vi "PH_GUI.set U32 ring GUI object.vi"(1 "Strings And Values [Empty]":T2, 2 "Ring Ref":refnum<vi>, 3 "Value":u32, 4 "Blinking (false)":bool, 5 "error in (no error)":errorcluster, 7 "Tip Strip [Empty]":string, 9 "Disabled (Enabled)":T1(ring), 11 "Visible (true)":bool=TRUE) -> (19 "error out":errorcluster)   [LabVIEW 2014, in "PH_Common.lvlib"]
doc: "Sets value and more for the referenced GUI object."
uses:
  <vilib>/Utility/miscctls.llb/LVStringsAndValuesArrayTypeDef_U32.ctl
  PH_Common.lvlib
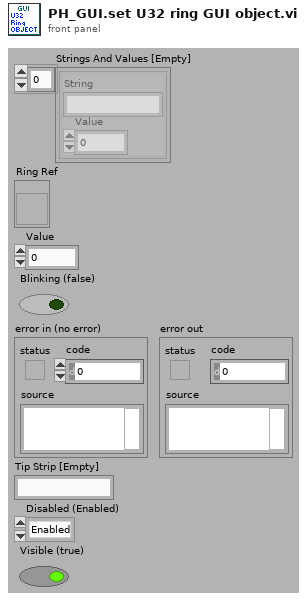
[diagram p1: front panel]
types:
  T1 = enum8{"Enabled", "Disabled", "Disabled and Grayed Out"}
  T2 = typedef "LVStringsAndValuesArrayTypeDef_U32.ctl" = cluster{"String":string, "Value":u32}[]
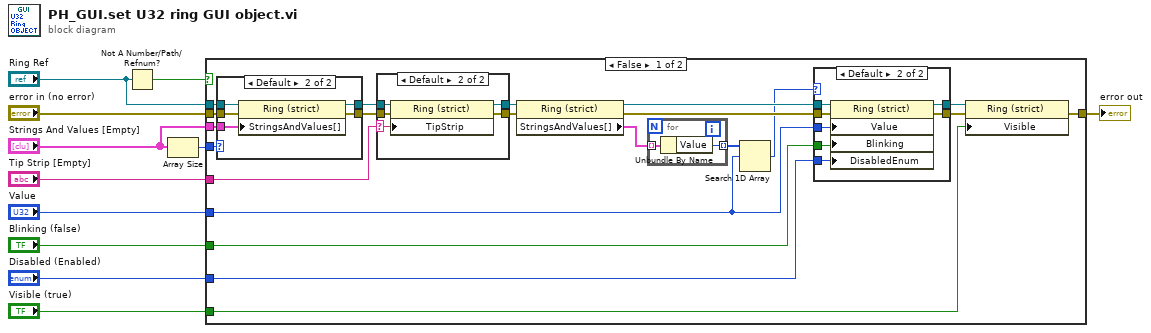
[diagram p0: block diagram]
diagram:
  n1 = Not A Number/Path/Refnum?(number/path/refnum="Ring Ref") -> (NaN/Path/Refnum?=w10:bool)
  n2 = Array Size(array="Strings And Values [Empty]") -> (size(s)=w5:i32)
  n3 = case shown="False" w10 {
    tunnel: "error in (no error)" -> [w24 w58]
    tunnel: "Ring Ref" -> [w25 _]
    tunnel: "Value" -> [w27 _]
    tunnel: "Blinking (false)" -> [w32 _]
    tunnel: [w15 w58] -> w7
    tunnel: w5 -> [w23 _]
    tunnel: "Strings And Values [Empty]" -> [w22 _]
    tunnel: "Tip Strip [Empty]" -> [w17 _]
    tunnel: "Disabled (Enabled)" -> [w16 _]
    tunnel: "Visible (true)" -> [w12 _]
    frame False {
      n4 = case shown="Default" w23 {
        tunnel: w25 -> [w41 w46]
        tunnel: [w41 w45] -> w21
        tunnel: w24 -> [w40 w44]
        tunnel: [w40 w43] -> w19
        tunnel: w22 -> [_ w42]
        frame 0 {
        }
        frame Default {
          n5 = property class="Ring (strict)"(reference=w46, error in=w44, "StringsAndValues[]"=w42) -> (reference out=w45:refnum<vi>, error out=w43:errorcluster)
        }
      }
      n6 = case shown="Default" w17 {
        selector: w17 -> [_ w35]
        tunnel: w21 -> [w34 w39]
        tunnel: [w34 w38] -> w20
        tunnel: w19 -> [w33 w37]
        tunnel: [w33 w36] -> w18
        frame "", "N/A" {
        }
        frame Default {
          n7 = property class="Ring (strict)"(reference=w39, error in=w37, "TipStrip"=w35) -> (reference out=w38:refnum<vi>, error out=w36:errorcluster)
        }
      }
      n8 = property class="Ring (strict)"(reference=w20, error in=w18) -> (reference out=w30:refnum<vi>, error out=w31:errorcluster, "StringsAndValues[]"=w29:T2)
      n9 = for {
        tunnel: w29 -> [w57] mode=indexing
        tunnel: [w56] -> w28 mode=indexing
        n10 = Unbundle By Name(w57) -> ("Value"=w56:u32)
      }
      n11 = Search 1D Array(1D array=w28, element=w27) -> (index of element=w26:i32)  [unwired: 1 in]
      n12 = case shown="Default" w26 {
        tunnel: [w48 w55] -> w14
        tunnel: w32 -> [_ w54]
        tunnel: w31 -> [w48 w53]
        tunnel: w30 -> [w47 w52]
        tunnel: w27 -> [_ w51]
        tunnel: w16 -> [_ w50]
        tunnel: [w47 w49] -> w13
        frame -1 {
        }
        frame Default {
          n13 = property class="Ring (strict)"(reference=w52, error in=w53, "Value"=w51, "Blinking"=w54, "DisabledEnum"=w50) -> (reference out=w49:refnum<vi>, error out=w55:errorcluster)
        }
      }
      n14 = property class="Ring (strict)"(reference=w13, error in=w14, "Visible"=w12) -> (error out=w15:errorcluster)  [unwired: 1 out]
    }
    frame True {
    }
  }
  "error out" <- w7
